vi "Control Drone.vi"(0 "UDP Output Port":refnum<k16>, 5 "Roll":sgl=-1.0, 7 "Pitch":sgl=-1.0, 9 "Yaw":sgl=-1.0, 11 "Veritical Speed":sgl=-1.0) -> (4 "UDP Output Port 2":refnum<k16>)   [LabVIEW 2011]
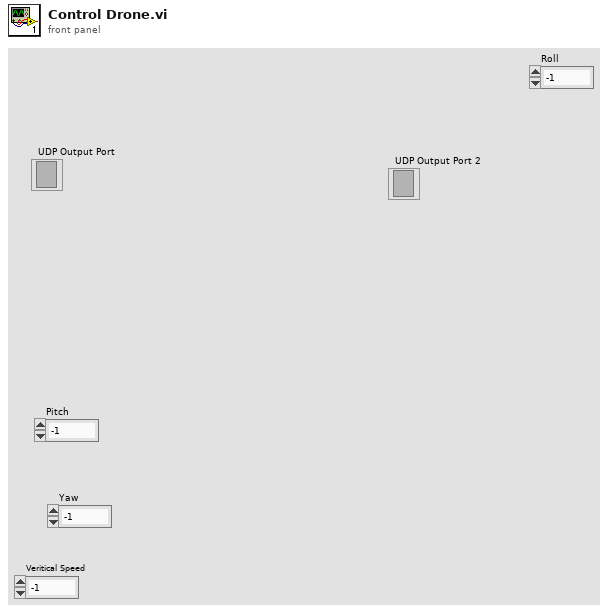
[diagram p1: front panel]
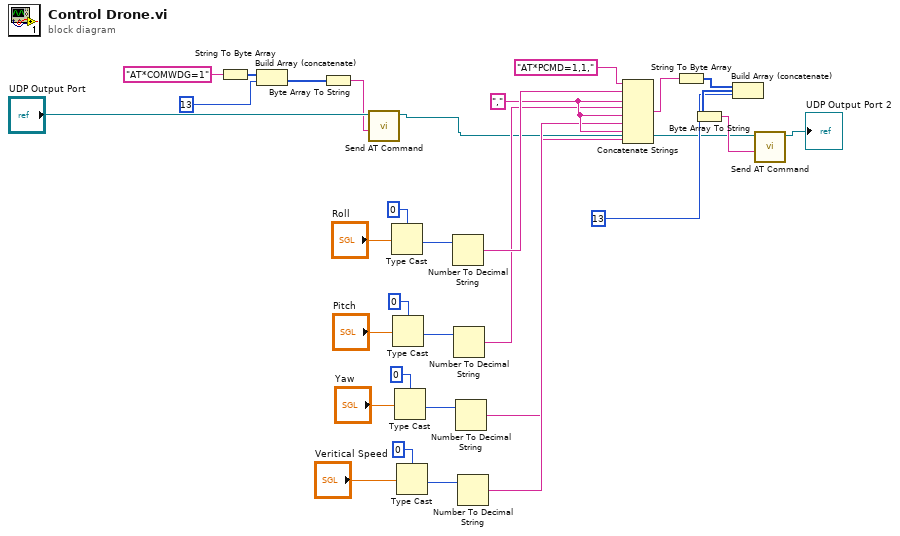
[diagram p0: block diagram]
diagram:
  w20 = ","
  n1 = String To Byte Array(string="AT*COMWDG=1") -> (unsigned byte array=w4:u8[])
  n2 = Build Array (concatenate)(w4, u8 13) -> (w1:u8[])
  n3 = Byte Array To String(unsigned byte array=w1) -> (string=w2:string)
  n4 = call "Send AT Command.vi"("AT Command"=w2, "UDP Output Port"="UDP Output Port") -> ("UDP Output Port"=w7:refnum<k16>)  [unwired: 9 in]
  n5 = Type Cast(type=u32 0, x="Roll") -> (*(type *) &x=w24:u32)
  n6 = Type Cast(type=u32 0, x="Pitch") -> (*(type *) &x=w17:u32)
  n7 = Type Cast(type=u32 0, x="Yaw") -> (*(type *) &x=w14:u32)
  n8 = Type Cast(type=u32 0, x="Veritical Speed") -> (*(type *) &x=w11:u32)
  n9 = Number To Decimal String(number=w24) -> (decimal integer string=w21:string)  [unwired: 1 in]
  n10 = Number To Decimal String(number=w17) -> (decimal integer string=w8:string)  [unwired: 1 in]
  n11 = Number To Decimal String(number=w14) -> (decimal integer string=w9:string)  [unwired: 1 in]
  n12 = Number To Decimal String(number=w11) -> (decimal integer string=w10:string)  [unwired: 1 in]
  n13 = Concatenate Strings("AT*PCMD=1,1,", w21, w20, w8, w20, w10, w20, w9) -> (w22:string)
  n14 = String To Byte Array(string=w22) -> (unsigned byte array=w30:u8[])
  n15 = Build Array (concatenate)(w30, u8 13) -> (w31:u8[])
  n16 = Byte Array To String(unsigned byte array=w31) -> (string=w28:string)
  n17 = call "Send AT Command.vi"("AT Command"=w28, "UDP Output Port"=w7) -> ("UDP Output Port"=→"UDP Output Port 2":refnum<k16>)  [unwired: 9 in]
